vi "Read ADCs.vi"() -> ()   [LabVIEW 2020, in "CTI-Visa-Scratchpad.lvlib"]
uses:
  CTI-Visa-Scratchpad.lvlib
  CTI-Visa/CTI-Visa.lvlib
  CTI-Visa-Pico/CTI-Visa-Pico.lvlib
panel:
  in  "Speed":i32(slide)=101 scale=1000.0..1.0
  in  "stop":bool
  out "ADC":dbl[][](graph)
  in  "Port":refnum<visa-resource-name>="COM3"
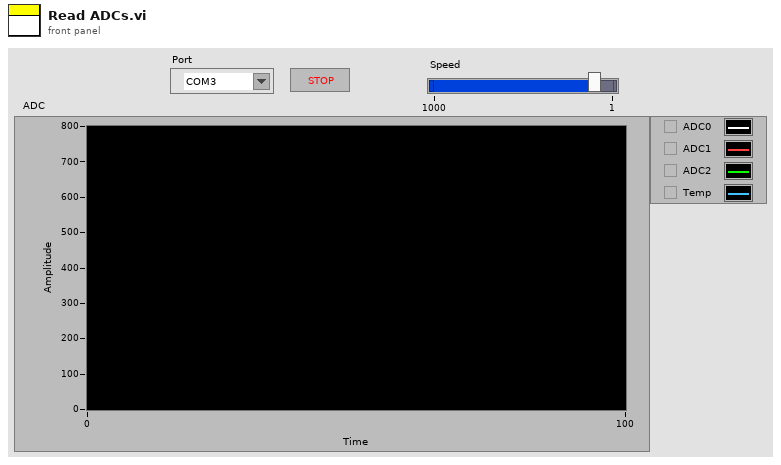
[diagram p1: front panel]
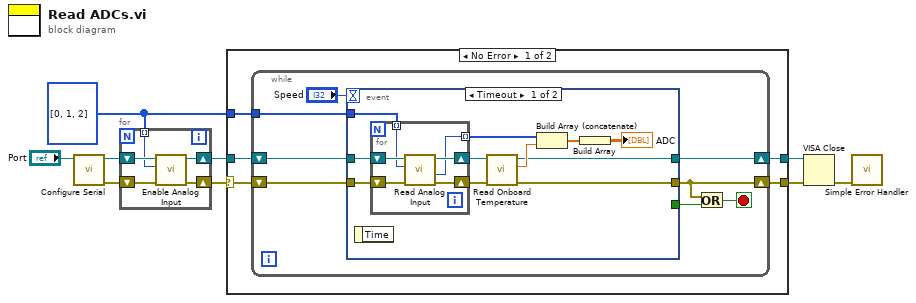
[diagram p0: block diagram]
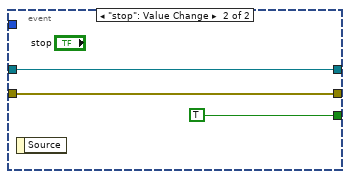
[diagram p2: hidden frame]
diagram:
  w4 = i32[] [0, 1, 2]
  n1 = call "Configure Serial.vi"("VISA resource name in"="Port") -> ("error out"=w7:errorcluster, "VISA resource name"=w8:refnum<visa-resource-name>)  [unwired: 9 in]
  n2 = for {
    shift-right: [w11] -> w5
    shift-left: w8 -> [w14]
    shift-right: [w10] -> w6
    shift-left: w7 -> [w13]
    tunnel: w4 -> [w12] mode=indexing
    n3 = call "Enable Analog Input.vi"("error in (no error)"=w13, "Channel"=w12, "VISA resource name in"=w14) -> ("error out"=w10:errorcluster, "VISA resource name"=w11:refnum<visa-resource-name>)  [unwired: 7 in]
  }
  n4 = case shown="No Error" w6 {
    selector: w6 -> [w17 w49]
    tunnel: w5 -> [w18 w48]
    tunnel: w4 -> [w19 _]
    tunnel: [w15 w49] -> w2
    tunnel: [w16 w48] -> w3
    frame No Error {
      n5 = while {
        tunnel: w19 -> [w26]
        shift-right: [w23] -> w16
        shift-left: w18 -> [w25]
        shift-right: [w22] -> w15
        shift-left: w17 -> [w24]
        stop <- w20 stop-if-true
        n6 = event shown="[0] Timeout" {
          selector: _ -> [_ _]
          dyn-events: _ -> [_ _]
          timeout: "Speed" -> [_ _]
          tunnel: w26 -> [w36 _]
          tunnel: w25 -> [w38 w45]
          tunnel: w24 -> [w37 w46]
          tunnel: [w29 w45] -> w23
          tunnel: [w28 w46] -> w22
          tunnel: [_ TRUE] -> w21
          event Timeout {
            n7 = event-data() -> ()  [unwired: 1 in, 1 out]
            n8 = for {
              shift-right: [w41] -> w34
              shift-left: w38 -> [w44]
              shift-right: [w40] -> w33
              shift-left: w37 -> [w43]
              tunnel: w36 -> [w42] mode=indexing
              tunnel: [w39] -> w32 mode=indexing
              n9 = call "Read Analog Input.vi"("error in (no error)"=w43, "Channel"=w42, "VISA resource name in"=w44) -> ("error out"=w40:errorcluster, "Value"=w39:u16, "VISA resource name"=w41:refnum<visa-resource-name>)  [unwired: 6 in]
            }
            n10 = call "Read Onboard Temperature.vi"("error in (no error)"=w33, "VISA resource name in"=w34) -> ("error out"=w28:errorcluster, "Temp degC"=w31:dbl, "VISA resource name"=w29:refnum<visa-resource-name>)  [unwired: 7 in]
            n11 = Build Array (concatenate)(w32, w31) -> (w30:dbl[])
            n12 = Build Array(w30) -> (→"ADC":dbl[][])
          }
          event "stop": Value Change {
            n13 = event-data() -> ()  [unwired: 1 in, 1 out]
          }
        }
        n14 = Or(x=w22, y=w21) -> (x .or. y?=w20:bool)
      }
    }
    frame Error {
    }
  }
  n15 = VISA Close(VISA resource name=w3, error in (no error)=w2) -> (error out=w1:errorcluster)
  n16 = call <vilib>:"Simple Error Handler.vi"("error in (no error)"=w1) -> ()  [unwired: 4 in, 5 out]
